vi "LVDimInterface.application example serv buffer.vi"() -> ()   [LabVIEW 2014, in "LVDimInterface.lvlib"]
doc: "This VI implements a DIM server, that publishes a loop counter as a DIM service"
uses:
  LVDimInterface.lvlib
panel:
  out "error out":errorcluster
  in  "update interval [ms]":u32=250
  out "loopCounter":i32
  in  "serverName":string="test28"
  in  "stop":bool
  in  "serviceName":string="testService"
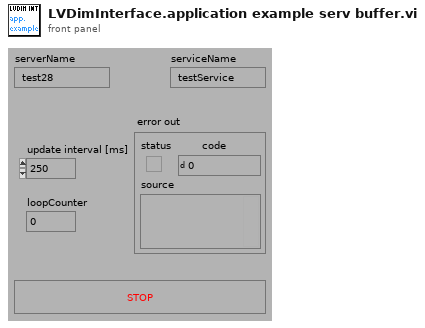
[diagram p1: front panel]
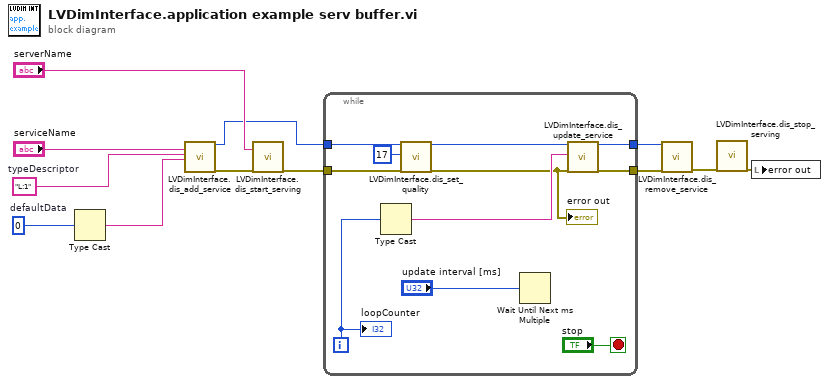
[diagram p0: block diagram]
diagram:
  w7 = 0  # defaultData
  w4 = "L:1"  # typeDescriptor
  n1 = Type Cast(x=w7) -> (*(type *) &x=w6:string)  [unwired: 1 in]
  n2 = call "LVDimInterface.dis_add_service.vi"("serviceName"="serviceName", "typeDescriptor"=w4, "data"=w6) -> ("my_serviceID"=w3:i32, "error out"=w11:errorcluster)  [unwired: 15 in]
  n3 = call "LVDimInterface.dis_start_serving.vi"("serverName"="serverName", "error in (no error)"=w11) -> ("error out"=w9:errorcluster)  [unwired: 16 in, 1 out]
  n4 = while {
    tunnel: [w21] -> w12
    tunnel: w9 -> [w19]
    tunnel: [w18] -> w2
    tunnel: w3 -> [w15]
    i -> [w20]
    stop <- "stop" stop-if-true
    n5 = Type Cast(x=w20) -> (*(type *) &x=w17:string)  [unwired: 1 in]
    n6 = call "LVDimInterface.dis_set_quality.vi"("my_serviceID"=w15, "quality"=17, "error in (no error)"=w19) -> ("my_serviceID (out)"=w14:i32, "error out"=w13:errorcluster)  [unwired: 15 in]
    "error out" <- w13
    n7 = Wait Until Next ms Multiple(millisecond multiple="update interval [ms]") -> ()  [unwired: 1 out]
    n8 = call "LVDimInterface.dis_update_service.vi"("my_serviceID"=w14, "data"=w17, "error in (no error)"=w13) -> ("my_serviceID out"=w21:i32, "error out"=w18:errorcluster)  [unwired: 14 in, 1 out]
    "loopCounter" <- w20
  }
  n9 = call "LVDimInterface.dis_remove_service.vi"("my_serviceID"=w12, "error in (no error)"=w2) -> ("error out"=w8:errorcluster)  [unwired: 17 in]
  n10 = call "LVDimInterface.dis_stop_serving.vi"("error in (no error)"=w8) -> ("error out"=w1:errorcluster)  [unwired: 18 in]
  n11 = local write "error out"(w1) -> ()
